vi "Add_AI_Task_#.vi"(8 "error in (no error)":errorcluster, 11 "DAQmxTaksContainer_General in":refnum<class "DAQmxTaksContainer_General.lvclass">) -> (0 "error out":errorcluster, 3 "DAQmxTaksContainer_General out":refnum<class "DAQmxTaksContainer_General.lvclass">)   [LabVIEW 2019, in "DAQmxTaksContainer_General.lvclass"]
uses:
  DAQmxTaksContainer_General.lvclass
  DAQmxTaksContainer_General.lvclass/DAQmxTaksContainer_General.ctl
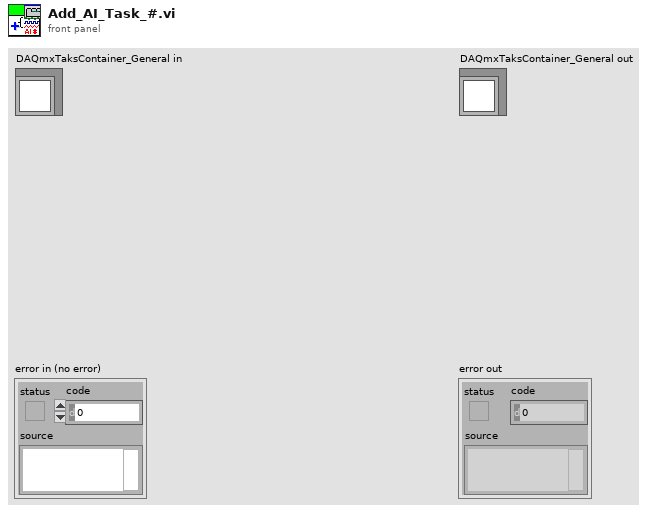
[diagram p1: front panel]
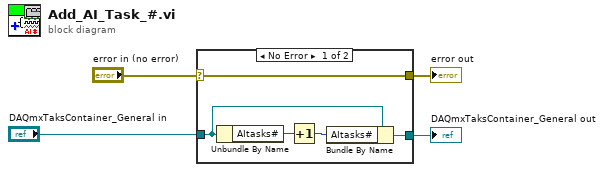
[diagram p0: block diagram]
diagram:
  n1 = case shown="No Error" "error in (no error)" {
    selector: "error in (no error)" -> [w9 w11]
    tunnel: [w9 w11] -> w3
    tunnel: [w5 w10] -> w1
    tunnel: "DAQmxTaksContainer_General in" -> [w8 w10]
    frame No Error {
      n2 = Unbundle By Name(w8) -> ("AItasks#"=w7:i32)
      n3 = Increment(x=w7) -> (x+1=w6:i32)
      n4 = Bundle By Name(cluster=w8, "AItasks#"=w6) -> (w5:refnum<class "DAQmxTaksContainer_General.lvclass">)
    }
    frame Error {
    }
  }
  "error out" <- w3
  "DAQmxTaksContainer_General out" <- w1
